vi "Main.vi"(7 "error in (no error)":errorcluster, 10 "ModuleAdmin":refnum<class "ModuleAdmin.lvclass">) -> ()   [LabVIEW 2018, in "AcPwrPlugins.lvlib"]
doc: "This VI is the critical engine of the AcPwr Plugin. It makes all the initialize, configure, and etc calls to the instrument drivers using their specifica API functions based upon the loaded configuration file."
uses:
  AcPwrPlugins/AcPwrPlugins.lvlib
  <userlib>/NIST/ModuleAdminLib/ModuleAdmin/ModuleAdmin.lvclass
  C:/Program Files (x86)/National Instruments/LabVIEW 2018/user.lib/NIST/ModuleAdminLib/ModuleAdminBase/ModuleAdminBase.lvclass
  AcPwrPlugins/AcPwrBaseClass/AcPwrBase.lvclass
  C:/Program Files (x86)/National Instruments/LabVIEW 2018/user.lib/NIST/BaseClasses/BasePlugin_class/BasePlugin.lvclass
  PublicAPI/Arguments/Requests/clStopArgument.ctl
  <userlib>/NIST/ModuleAdminLib/ModuleAdmin/ModuleAdmin.lvclass/ModuleAdmin.ctl
  <userlib>/NIST/BaseClasses/BasePlugin_class/BasePlugin.lvclass/BasePlugin.ctl
  <vilib>/Utility/error.llb/DialogType.ctl
  <userlib>/NIST/ModuleAdminLib/ModuleAdmin/Accessors/Read ShowPanel_.vi
  <userlib>/NIST/ModuleAdminLib/ModuleAdmin/Accessors/Write ShowPanel_.vi
  <userlib>/NIST/BaseClasses/BasePlugin_class/Accessors/Write PluginIniFilePath.vi
  <userlib>/NIST/BaseClasses/BasePlugin_class/Accessors/Read PluginIniFilePath.vi
  <userlib>/NIST/ModuleAdminLib/ModuleAdmin/Accessors/Read CloneRegRef.vi
  <extravilib>/ChannelInstances/Tag-bool/Read With Abort.vi
  <extravilib>/ChannelInstances/Tag-bool/Write With Abort.vi
  <extravilib>/ChannelInstances/Tag-bool/Instantiate.vi
  <extravilib>/ChannelInstances/Tag-bool/EndpointRead.vi
  <vilib>/Utility/error.llb/Error Cluster From Error Code.vi
  <extravilib>/ChannelInstances/Tag-bool/Endpoint.vi
  <vilib>/ErrorRing/Error Ring.xnode
  <userlib>/NIST/ModuleAdminLib/CloneRegistration/CloneRegistration.lvclass
  AcPwrModule.lvlib
  <userlib>/NIST/BaseClasses/Object_class/BaseObject.lvclass
  <userlib>/NIST/ModuleAdminLib/ModuleAdmin.lvlib
  <extravilib>/ChannelInstances/Tag-bool.lvlib
panel:
  out "RunTime(ms)":u32
  out "error out":errorcluster
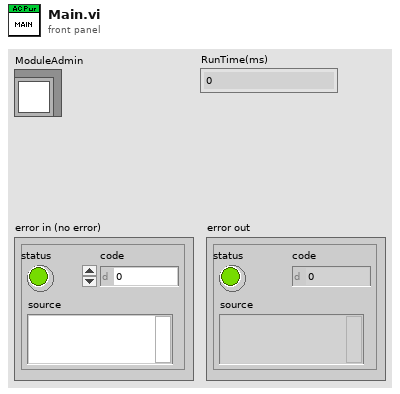
[diagram p1: front panel]
types:
  T1 = typedef "clRequestEvents.ctl" = cluster{"StopRequest":refnum<user-event>, "PathToINI":refnum<user-event>, " LoadPlugin":refnum<user-event>, "ShowPanel":refnum<user-event>, "PrefDlg":refnum<user-event>, "InitAcPwr":refnum<user-event>, "Reset":refnum<user-event>, "Close":refnum<user-event>, "StopMeas":refnum<user-event>, "StartMeas":refnum<user-event>, "ConfigDevice":refnum<user-event>, "DeviceOn":refnum<user-event>, "DeviceOff":refnum<user-event>, "GetSettings":refnum<user-event>, "SetSettings":refnum<user-event>}
  T2 = typedef "clBroadcastEvents.ctl" = cluster{"DidInit":refnum<user-event>, "StatusUpdate":refnum<user-event>, "ErrorReport":refnum<user-event>, "DidStop":refnum<user-event>, "PathToINI":refnum<user-event>, "Measurements":refnum<user-event>, "LoadConfigFile":refnum<user-event>, "GetSettings":refnum<user-event>, "SetSettings":refnum<user-event>, "GetType&ID":refnum<user-event>, "GotSettings":refnum<user-event>}
  T3 = typedef "clStopArgument.ctl" = cluster{"Exit via Stop Module Req?":bool, "Wait for Module to stop?":bool, "ModuleAdmin":refnum<class "ModuleAdmin.lvclass">}
  T4 = enum32{"Invalid", "Standard", "Closed", "Hidden", "Minimized", "Maximized"}
  T5 = typedef "Tag-bool.lvlib/))Channel.ctl" = refnum<queue>
  T6 = typedef "DialogType.ctl" = u16
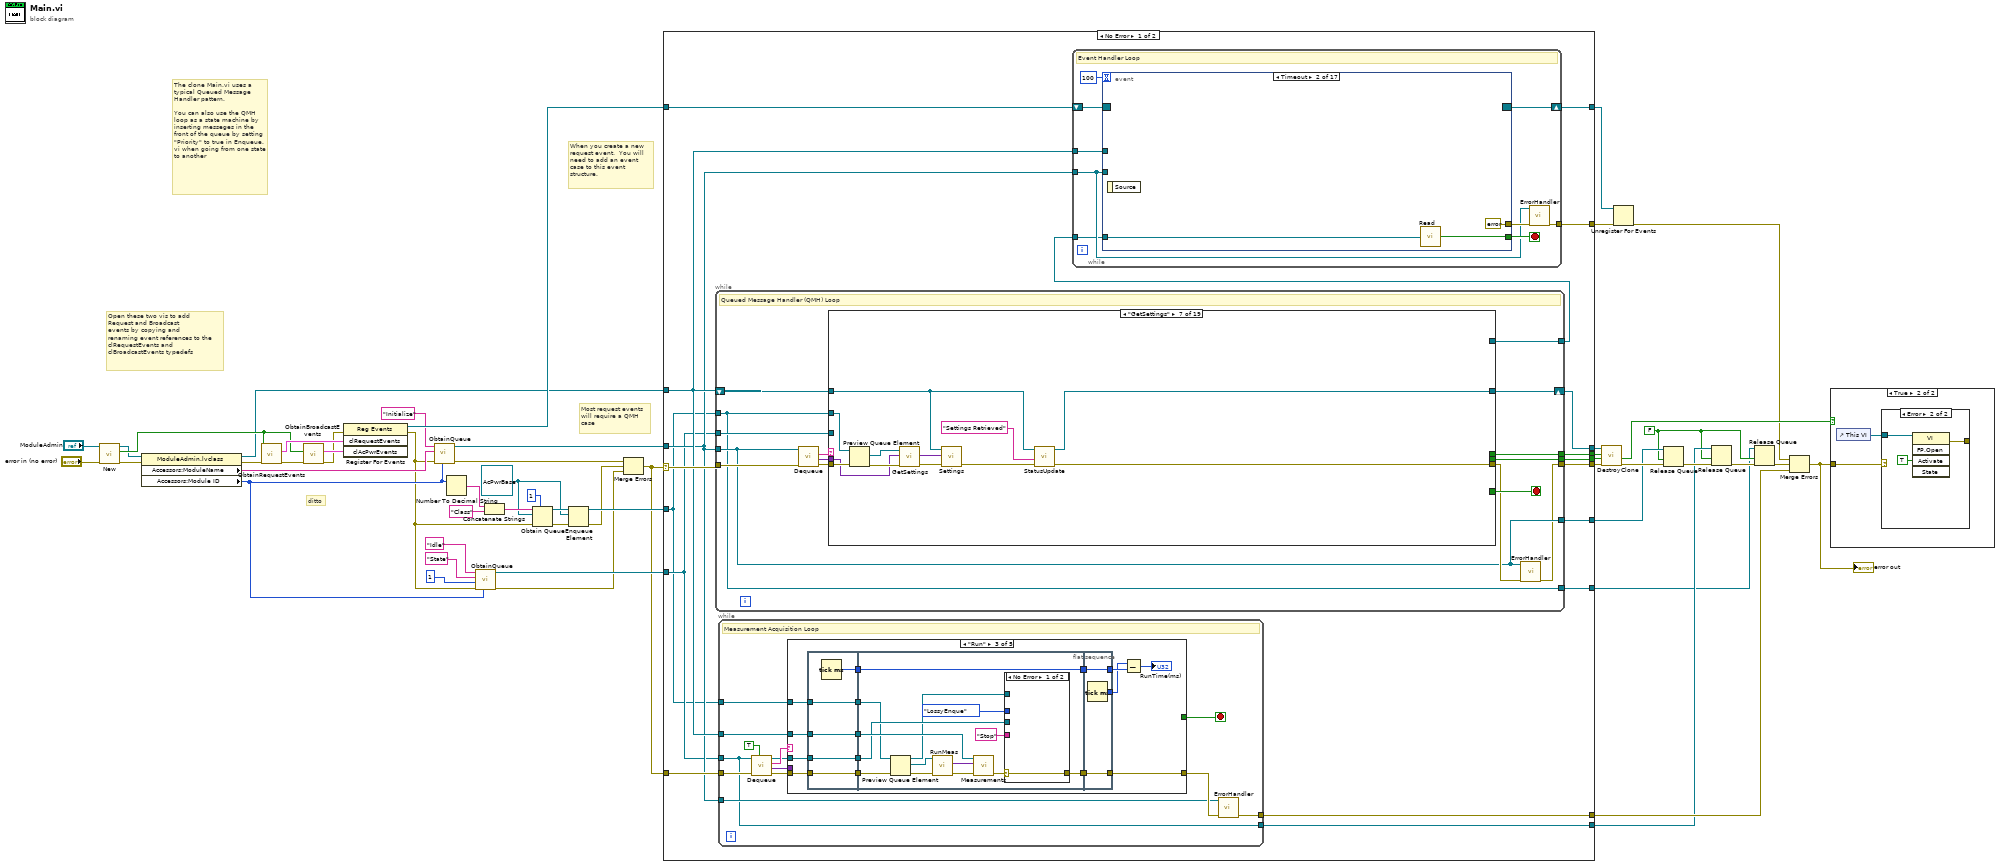
[diagram p0: block diagram]
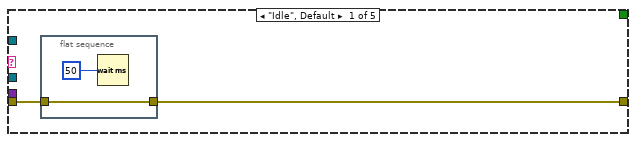
[diagram p2: hidden frame]
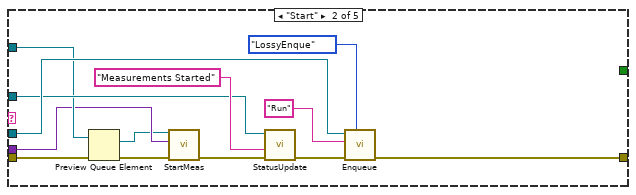
[diagram p3: hidden frame]
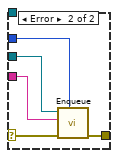
[diagram p4: hidden frame]
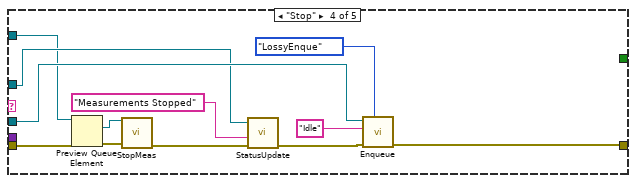
[diagram p5: hidden frame]
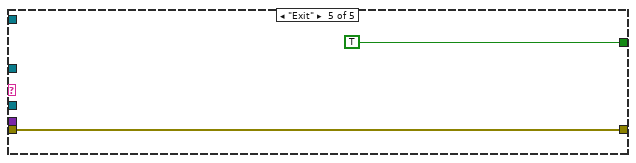
[diagram p6: hidden frame]
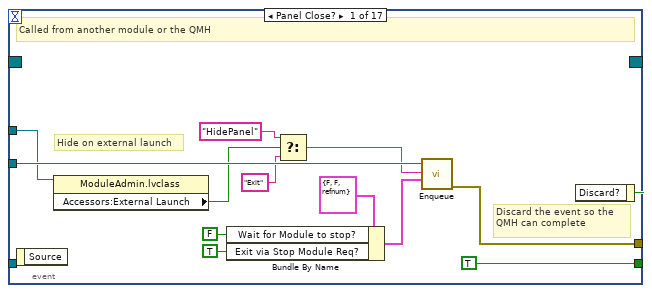
[diagram p7: hidden frame]
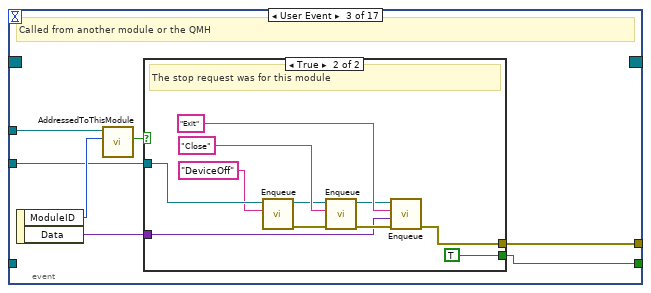
[diagram p8: hidden frame]
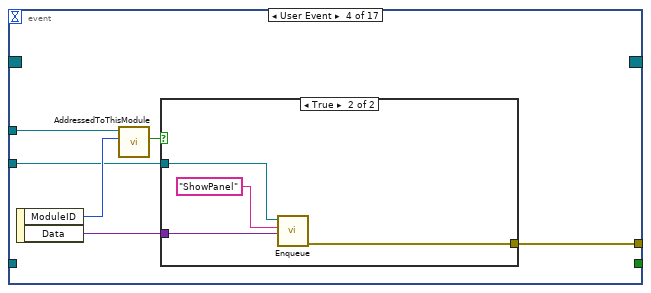
[diagram p10: hidden frame]
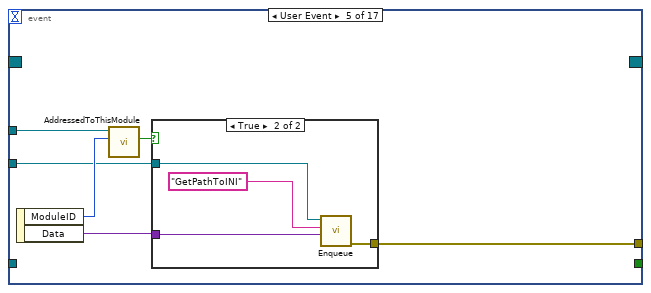
[diagram p12: hidden frame]
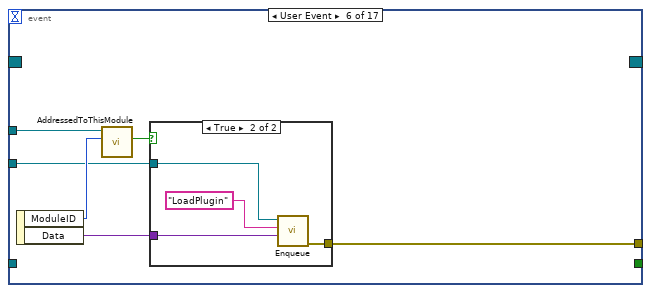
[diagram p14: hidden frame]
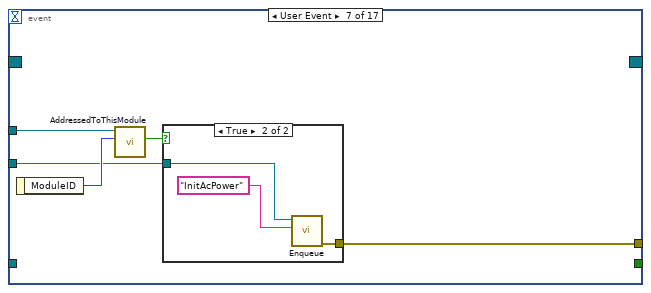
[diagram p16: hidden frame]
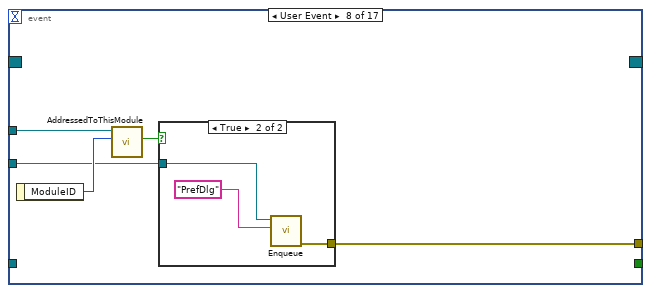
[diagram p18: hidden frame]
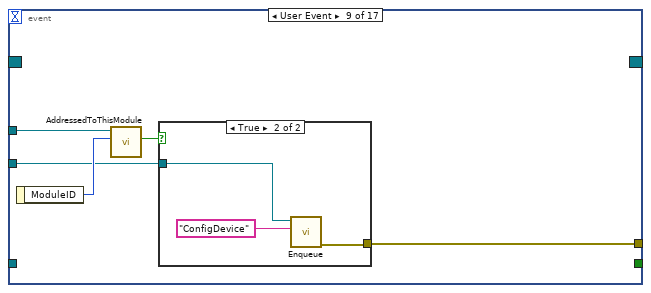
[diagram p20: hidden frame]
diagram:
  w13 = refnum<class "AcPwrBase.lvclass"> refnum ("MyPlugins.lvlib:MyPluginsBase.lvclass")
  w19 = FALSE ("force destroy? (F)")
  # "The clone Main.vi uses a typical Queued Message Handler pattern.  \n\nYou can also use the QMH loop as a state machine by inserting messeges in the front of the queue by setting \"Priority\" to true in Enqueue.vi when going from one state to another"
  # "Open these two vis to add\nRequest and Broadcast \nevents by copying and \nrenaming event references to the \nclRequestEvents and \nclBroadcastEvents typedefs"
  # "ditto"
  # "Most request events\nwill require a QMH\ncase"
  # "When you create a new request event.  You will need to add an event case to this event structure."
  n1 = call <userlib>:"New.vi"("error in (no error)"="error in (no error)", "ModuleAdmin"="ModuleAdmin") -> ("error out"=w33:errorcluster, "First?"=w47:bool, "ModuleAdmin"=w34:refnum<class "ModuleAdmin.lvclass">)  [unwired: 6 in, 1 out]
  n2 = property class="ModuleAdmin.lvclass"(reference=w34, error in=w33) -> (reference out=w30:refnum<class "ModuleAdmin.lvclass">, error out=w32:errorcluster, "Accessors:ModuleName"=w31:string, "Accessors:Module ID"=w23:i32)
  n3 = call "ObtainRequestEvents.vi"("error in (no error)"=w32, "CreateNew (F)"=w47) -> ("error out"=w46:errorcluster, "clRequestEvents"=w49:T1)  [unwired: 8 in]
  n4 = call "ObtainBroadcastEvents.vi"("error in (no error)"=w46, "CreateNew? (F)"=w47) -> ("error out"=w12:errorcluster, "clAcPwrEvents"=w45:T2)  [unwired: 8 in]
  n5 = register-events(error in=w12, w49, w45) -> (reference out=w44:refnum<event-registration>, error out=w11:errorcluster)  [unwired: 1 in]
  n6 = call "ObtainQueue.vi"("ModuleID"=w23, "error in (no error)"=w11, "ModuleName"=w31, "Initial Message"="Initialize" ("ModuleName")) -> ("error out"=w7:errorcluster, "MessageQueue"=w48:refnum<queue>)  [unwired: 6 in]
  n7 = Number To Decimal String(number=w23) -> (decimal integer string=w24:string)  [unwired: 1 in]
  n8 = call "ObtainQueue.vi"("ModuleID"=w23, "error in (no error)"=w11, "max queue size (-1, unlimited)"=1, "ModuleName"="State", "Initial Message"="Idle") -> ("error out"=w5:errorcluster, "MessageQueue"=w28:refnum<queue>)  [unwired: 5 in]
  n9 = Concatenate Strings(w24, "Class" ("ModuleName")) -> (w21:string)
  n10 = Obtain Queue(max queue size (-1, unlimited)=1, name (unnamed)=w21, element data type=w13, error in (no error)=w11) -> (queue out=w15:refnum<queue>, error out=w20:errorcluster)  [unwired: 1 in, 1 out]
  n11 = Enqueue Element(queue=w15, element=w13, error in (no error)=w20) -> (queue out=w14:refnum<queue>, error out=w6:errorcluster)  [unwired: 1 in, 1 out]
  n12 = Merge Errors(w7, w6, w5) -> (w4:errorcluster)
  n13 = case shown="No Error" w4 {
    selector: w4 -> [w69 w920]
    tunnel: w48 -> [w57 w913]
    tunnel: w30 -> [w58 w918]
    tunnel: [w68 w909] -> w1
    tunnel: w44 -> [w67 w914]
    tunnel: [w66 w917] -> w2
    tunnel: [w65 _] -> w42
    tunnel: [w64 _] -> w41
    tunnel: [w63 w909] -> w39
    tunnel: [w62 w914] -> w38
    tunnel: [w61 w913] -> w35
    tunnel: w4 -> [w60 w912]
    tunnel: [w59 w912] -> w29
    tunnel: w28 -> [w55 w911]
    tunnel: [w56 w911] -> w26
    tunnel: w14 -> [w54 w910]
    tunnel: [w53 w910] -> w16
    frame No Error {
      n14 = while {
        tunnel: w57 -> [w339]
        tunnel: w69 -> [w348]
        tunnel: [w338] -> w68
        tunnel: [w343] -> w65
        tunnel: [w342] -> w64
        shift-right: [w340] -> w66
        shift-left: w58 -> [w344]
        tunnel: [w339] -> w61
        tunnel: w55 -> [w337]
        tunnel: w54 -> [w336]
        tunnel: [w336] -> w53
        tunnel: [w335] -> w52
        stop <- w349 stop-if-true
        # "Queued Message Handler (QMH) Loop"
        n15 = call "Dequeue.vi"("error in (no error)"=w348, "MessageQueue"=w339) -> ("error out"=w347:errorcluster, "Message Data"=w345:variant, "Message"=w346:string)  [unwired: 5 in, 2 out]
        n16 = case shown="\"GetSettings\"" w346 {
          selector: w346 -> [_ _ _ _ _ _ _ _ _ _ _ _ _ _ _ _ _ _ w897]
          tunnel: [_ _ _ _ _ _ _ _ _ _ _ _ _ _ _ _ w857 _ _] -> w349
          tunnel: w344 -> [w371 w388 w395 w447 w460 w491 w533 w556 w611 w620 w668 w715 w721 w731 w826 w849 w860 w874 w900]
          tunnel: [w360 w382 w396 w448 w459 w490 w539 w555 w601 w622 w671 w716 w722 w732 w828 w850 w868 w875 w892] -> w341
          tunnel: w347 -> [w353 w391 w405 w442 w456 w489 w543 w554 w607 w618 w667 w717 w723 w727 w815 w837 w864 w872 _]
          tunnel: w345 -> [_ w390 w407 _ _ _ w532 w544 _ _ _ w711 _ _ _ _ w861 w882 _]
          tunnel: [_ _ _ _ _ _ _ _ _ _ _ _ _ _ _ _ w866 _ _] -> w343
          tunnel: [_ _ _ _ _ _ _ _ _ _ _ _ _ _ _ _ w865 _ _] -> w342
          tunnel: [w354 w387 w393 w446 w458 w486 w537 w551 w600 w619 w669 w715 w721 w730 w825 w848 w860 w873 w895] -> w340
          tunnel: w337 -> [_ _ _ _ w454 w485 _ w550 w599 w621 w670 w714 w720 w728 w813 w840 w862 _ _]
          tunnel: w336 -> [_ _ w392 w440 w453 w488 w542 w553 _ w617 w666 _ _ w724 w816 w835 _ _ _]
          tunnel: [_ _ _ _ _ _ _ _ _ _ _ _ _ _ _ _ w856 w871 _] -> w335
          frame "Initialize" {
            # "After the QMH, Class, and State Queue have been created this loop enters the intialize phase."
            n17 = property class="ModuleAdmin.lvclass"(reference=w371, error in=w353) -> (reference out=w358:refnum<class "ModuleAdmin.lvclass">, error out=w368:errorcluster, "Accessors:ShowPanel_"=w357:bool, "Accessors:External Launch"=w356:bool, "Accessors:Module ID"=w351:i32, "Accessors:ModuleName"=w352:string)
            n18 = Compound Arithmetic op=OR(w357, invert w356) -> (w355:bool)
            n19 = Select(t=T4."Standard" ("Front Panel Window:State"), s=w355, f=T4."Hidden" ("Front Panel Window:State")) -> (s? t:f=w364:T4)
            n20 = invoke class="VI" method="FP.Open"(error in=w368, "State"=w364) -> (reference out=w350:refnum<vi>, error out=w367:errorcluster)  [unwired: 3 in, 3 out]
            n21 = call <userlib>:"ModuleName.vi"("Name"=w352, "ModuleID"=w351) -> ("ModuleName"=w363:string)  [unwired: 9 in]
            n22 = property class="VI"(reference=w350, error in=w367, "Front Panel.Title"=w363) -> (reference out=w370:refnum<vi>, error out=w369:errorcluster)
            n23 = invoke class="VI" method="FP.Center"(reference=w370, error in=w369) -> (error out=w359:errorcluster)  [unwired: 1 in, 2 out]
            n24 = case shown="True" w356 {
              tunnel: [w372 w378] -> w361
              tunnel: [w373 w375] -> w354
              tunnel: w359 -> [w372 w377]
              tunnel: w358 -> [w373 w374]
              frame False {
              }
              frame True {
                n25 = call <userlib>:"WaitOnModuleSync.vi"("error in (no error)"=w377, "ModuleAdmin"=w374) -> ("error out"=w379:errorcluster, "ModuleAdmin"=w376:refnum<class "ModuleAdmin.lvclass">)  [unwired: 8 in]
                n26 = call <userlib>:"WaitOnEventSync.vi"("error in (no error)"=w379, "ModuleAdmin"=w376) -> ("error out"=w378:errorcluster, "ModuleAdmin"=w375:refnum<class "ModuleAdmin.lvclass">)  [unwired: 8 in]
              }
            }
            n27 = call "DidInit.vi"("Init?"=TRUE, "error in (no error)"=w361, "ModuleAdmin"=w354) -> ("error out"=w360:errorcluster)  [unwired: 8 in]
          }
          frame "ShowPanel" {
            # "The front panel can be shown or hidden"
            n28 = Variant To Data(error in=w391, type=TRUE, Variant=w390) -> (data=w384:bool, error out=w381:errorcluster)
            n29 = property class="ModuleAdmin.lvclass"(reference=w388, error in=w381, "Accessors:ShowPanel_"=w384) -> (reference out=w387:refnum<class "ModuleAdmin.lvclass">, error out=w380:errorcluster)
            n30 = Select(t=T4."Standard" ("Front Panel Window:State"), s=w384, f=T4."Hidden" ("Front Panel Window:State")) -> (s? t:f=w383:T4)
            n31 = property class="VI"(error in=w380, "FP.State"=w383) -> (error out=w382:errorcluster)  [unwired: 1 in, 1 out]
          }
          frame "LoadPlugin" {
            # "Dynamically oads and initializes a plugin from the .ini file"
            n32 = Variant To Data(error in=w405, type=path "", Variant=w407) -> (data=w394:path, error out=w404:errorcluster)
            n33 = Current VI's Path() -> (path=w402:path)
            n34 = call <userlib>:"GetPathToClass.vi"("error in (no error)"=w404, "configuration file path"=w394) -> ("error IO"=w400:errorcluster, "PathToClass"=w403:path)  [unwired: 8 in]
            n35 = Build Path(base path=w402, name or relative path=w403) -> (appended path=w401:path)
            n36 = call <vilib>:"Check if File or Folder Exists.vi"("error in (no error)"=w400, "path"=w401) -> ("error out"=w397:errorcluster, "file or folder exists?"=w399:bool, "dup path"=w398:path)  [unwired: 7 in]
            n37 = case shown="False" w399 {
              tunnel: w398 -> [w410 w419]
              tunnel: w397 -> [_ w426]
              tunnel: [w409 w436] -> w396
              tunnel: w395 -> [w408 w432]
              tunnel: w394 -> [_ w433]
              tunnel: [w408 w431] -> w393
              tunnel: w392 -> [_ w424]
              frame False {
                n38 = Path To String(path=w410) -> (string=w411:string)
                n39 = xnode "Error Ring"("parameter 0"=w411) -> ("error out"=w409:errorcluster)
              }
              frame True {
                (unwired) refnum<class "AcPwrBase.lvclass"> refnum ("MyPlugins.lvlib:MyPluginsBase.lvclass")
                n40 = Strip Path(path=w419) -> (name=w422:string)  [unwired: 1 out]
                n41 = Preview Queue Element(queue=w424, error in (no error)=w426) -> (element=w423:refnum<class "AcPwrBase.lvclass">, error out=w425:errorcluster)  [unwired: 1 in, 2 out]
                n42 = call-dynamic "LoadClassFromFile.vi"("error in (no error)"=w425, "class path"=w419, "reference in"=w423) -> ("error out"=w434:errorcluster, "reference out"=w435:refnum<class "AcPwrBase.lvclass">)  [unwired: 7 in]
                n43 = property class="AcPwrBase.lvclass"(reference=w435, error in=w434, "Accessors:PluginIniFilePath"=w433) -> (reference out=w430:refnum<class "AcPwrBase.lvclass">, error out=w429:errorcluster)
                n44 = call-dynamic "DefaultFromIni.vi"("error in (no error)"=w429, "AcPwrBase"=w430) -> ("error out"=w427:errorcluster, "AcPwrBase"=w428:refnum<class "AcPwrBase.lvclass">)  [unwired: 8 in]
                n45 = Lossy Enqueue Element(queue=w424, element=w428, error in (no error)=w427) -> (error out=w420:errorcluster)  [unwired: 3 out]
                n46 = Format Into String(format string="Plugin %s loaded ", error in=w420, w422) -> (resulting string=w437:string, error out=w421:errorcluster)  [unwired: 1 in]
                n47 = call "StatusUpdate.vi"("error in (no error)"=w421, "Status"=w437, "Module"=w432) -> ("error out"=w436:errorcluster, "Module"=w431:refnum<class "ModuleAdmin.lvclass">)  [unwired: 7 in]
              }
            }
          }
          frame "GetPathToINI" {
            # "Broadcast the path to the .ini file"
            n48 = Preview Queue Element(queue=w440, error in (no error)=w442) -> (element=w445:refnum<class "AcPwrBase.lvclass">, error out=w441:errorcluster)  [unwired: 1 in, 2 out]
            n49 = property class="AcPwrBase.lvclass"(reference=w445, error in=w441) -> (error out=w444:errorcluster, "Accessors:PluginIniFilePath"=w439:path)  [unwired: 1 out]
            n50 = property class="ModuleAdmin.lvclass"(reference=w447, error in=w444) -> (reference out=w446:refnum<class "ModuleAdmin.lvclass">, error out=w443:errorcluster, "Accessors:Module ID"=w449:i32)
            n51 = call "PathToINIBroadcast.vi"("error in (no error)"=w443, "PathToINI"=w439, "ModuleID"=w449) -> ("error out"=w448:errorcluster)  [unwired: 8 in]
          }
          frame "InitAcPower" {
            n52 = call "Dequeue.vi"("PreviewQueue(F)"=TRUE, "error in (no error)"=w456, "MessageQueue"=w454) -> ("error out"=w455:errorcluster, "Message"=w451:string)  [unwired: 4 in, 3 out]
            n53 = Equal?(x="Run" ("y"), y=w451) -> (x = y?=w457:bool)
            n54 = case shown="False" w457 {
              tunnel: w460 -> [w472 w474]
              tunnel: [w471 w473] -> w459
              tunnel: [w469 w474] -> w458
              tunnel: w455 -> [w466 _]
              tunnel: w453 -> [w464 _]
              frame False {
                n55 = Preview Queue Element(queue=w464, error in (no error)=w466) -> (queue out=w462:refnum<queue>, element=w468:refnum<class "AcPwrBase.lvclass">, error out=w465:errorcluster)  [unwired: 1 in, 1 out]
                n56 = call-dynamic "Initialize.vi"("error in (no error)"=w465, "AcPwrBase in"=w468) -> ("error out"=w463:errorcluster, "AcPwrBase out"=w467:refnum<class "AcPwrBase.lvclass">)  [unwired: 8 in]
                n57 = Lossy Enqueue Element(queue=w462, element=w467, error in (no error)=w463) -> (error out=w461:errorcluster)  [unwired: 3 out]
                n58 = call "StatusUpdate.vi"("error in (no error)"=w461, "Status"="Device Initialized", "Module"=w472) -> ("error out"=w471:errorcluster, "Module"=w469:refnum<class "ModuleAdmin.lvclass">)  [unwired: 7 in]
              }
              frame True {
                n59 = xnode "Error Ring"() -> ("error out"=w473:errorcluster)
              }
            }
          }
          frame "ConfigDevice" {
            n60 = Preview Queue Element(queue=w488, error in (no error)=w489) -> (queue out=w487:refnum<queue>, element=w483:refnum<class "AcPwrBase.lvclass">, error out=w484:errorcluster)  [unwired: 1 in, 1 out]
            n61 = call-dynamic "ChangeWhileMeasuring.vi"("error in (no error)"=w484, "AcPwrBase in"=w483) -> ("error out"=w482:errorcluster, "OutputOrLoadValue"=w480:bool, "AcPwrBase out"=w481:refnum<class "AcPwrBase.lvclass">)  [unwired: 6 in, 1 out]
            n62 = case shown="True" w480 {
              tunnel: w491 -> [w501 w526]
              tunnel: w481 -> [w499 w508]
              tunnel: [w498 w518] -> w490
              tunnel: w482 -> [w497 w511]
              tunnel: w487 -> [w493 w515]
              tunnel: [w496 w514] -> w486
              tunnel: w485 -> [_ w510]
              frame True {
                n63 = call-dynamic "ConfigDevice.vi"("error in (no error)"=w497, "AcPwrBase in"=w499) -> ("error out"=w495:errorcluster, "AcPwrBase out"=w492:refnum<class "AcPwrBase.lvclass">)  [unwired: 8 in]
                n64 = Lossy Enqueue Element(queue=w493, element=w492, error in (no error)=w495) -> (error out=w494:errorcluster)  [unwired: 3 out]
                n65 = call "StatusUpdate.vi"("error in (no error)"=w494, "Status"="Device Configured", "Module"=w501) -> ("error out"=w498:errorcluster, "Module"=w496:refnum<class "ModuleAdmin.lvclass">)  [unwired: 7 in]
              }
              frame False {
                w523 = TRUE ("OverwriteClass? (F)")
                n66 = call "Dequeue.vi"("PreviewQueue(F)"=TRUE, "error in (no error)"=w511, "MessageQueue"=w510) -> ("error out"=w509:errorcluster, "Message"=w503:string, "MessageQueue"=w502:refnum<queue>)  [unwired: 4 in, 2 out]
                n67 = Equal?(x="Run" ("y"), y=w503) -> (x = y?=w506:bool)
                n68 = call "CheckonIdle.vi"("MessageQueue"=w502, "OverwriteClass? (F)"=w523, "error in (no error)"=w509, "ChangeOccured? (F)"=w523, "AcPwrBase in"=w508) -> ("Error Out"=w524:errorcluster, "Write?"=w520:bool, "AcPwrBase out"=w522:refnum<class "AcPwrBase.lvclass">)  [unwired: 4 in]
                n69 = call-dynamic "ConfigDevice.vi"("error in (no error)"=w524, "AcPwrBase in"=w522) -> ("error out"=w517:errorcluster, "AcPwrBase out"=w521:refnum<class "AcPwrBase.lvclass">)  [unwired: 8 in]
                n70 = case shown="True" w520 {
                  tunnel: [w527 w531] -> w516
                  tunnel: w517 -> [w527 w530]
                  tunnel: w515 -> [_ w529]
                  tunnel: w521 -> [_ w528]
                  frame False {
                  }
                  frame True {
                    n71 = Lossy Enqueue Element(queue=w529, element=w528, error in (no error)=w530) -> (error out=w531:errorcluster)  [unwired: 3 out]
                  }
                }
                n72 = call "StatusUpdate.vi"("error in (no error)"=w516, "Status"="Device Configured", "Module"=w526) -> ("error out"=w519:errorcluster, "Module"=w514:refnum<class "ModuleAdmin.lvclass">)  [unwired: 7 in]
                n73 = Select(t="Start" ("strngStateIn"), s=w506, f=w503) -> (s? t:f=w504:string)
                n74 = call "Enqueue.vi"("EnqueType (Enque)"=enum16{"LossyEnque", "EnqueAtFront", "Enque"}."LossyEnque" ("Enum"), "error in (no error)"=w519, "Message"=w504, "MessageQueue"=w502) -> ("error out"=w518:errorcluster)  [unwired: 6 in, 1 out]
              }
            }
          }
          frame "GetSettings" {
            n75 = Preview Queue Element(queue=w542, error in (no error)=w543) -> (element=w540:refnum<class "AcPwrBase.lvclass">, error out=w541:errorcluster)  [unwired: 1 in, 2 out]
            n76 = call-dynamic "GetSettings.vi"("error in (no error)"=w541, "SettingsToRetrieve"=w532, "AcPwrBase in"=w540) -> ("error out"=w536:errorcluster, "RetrievedSettings"=w534:variant)  [unwired: 6 in, 1 out]
            n77 = call "Settings.vi"("error in (no error)"=w536, "variant"=w534, "Module"=w533) -> ("error out"=w535:errorcluster)  [unwired: 8 in]
            n78 = call "StatusUpdate.vi"("error in (no error)"=w535, "Status"="Settings Retrieved", "Module"=w533) -> ("error out"=w539:errorcluster, "Module"=w537:refnum<class "ModuleAdmin.lvclass">)  [unwired: 7 in]
          }
          frame "SetSettings" {
            n79 = Preview Queue Element(queue=w553, error in (no error)=w554) -> (queue out=w552:refnum<queue>, element=w548:refnum<class "AcPwrBase.lvclass">, error out=w549:errorcluster)  [unwired: 1 in, 1 out]
            n80 = call-dynamic "ChangeWhileMeasuring.vi"("error in (no error)"=w549, "AcPwrBase in"=w548) -> ("error out"=w547:errorcluster, "OutputOrLoadValue"=w545:bool, "AcPwrBase out"=w546:refnum<class "AcPwrBase.lvclass">)  [unwired: 6 in, 1 out]
            n81 = case shown="True" w545 {
              tunnel: w556 -> [w567 w593]
              tunnel: w546 -> [w560 w570]
              tunnel: [w565 w588] -> w555
              tunnel: w547 -> [w561 w582]
              tunnel: w552 -> [w562 w586]
              tunnel: [w564 w585] -> w551
              tunnel: w550 -> [_ w581]
              tunnel: w544 -> [w559 w571]
              frame True {
                n82 = call-dynamic "SetSettings.vi"("error in (no error)"=w561, "Variant"=w559, "AcPwrBase in"=w560) -> ("error out"=w557:errorcluster, "AcPwrBase Out"=w558:refnum<class "AcPwrBase.lvclass">)  [unwired: 7 in]
                n83 = Lossy Enqueue Element(queue=w562, element=w558, error in (no error)=w557) -> (error out=w563:errorcluster)  [unwired: 3 out]
                n84 = call "StatusUpdate.vi"("error in (no error)"=w563, "Status"="Settings Set", "Module"=w567) -> ("error out"=w565:errorcluster, "Module"=w564:refnum<class "ModuleAdmin.lvclass">)  [unwired: 7 in]
              }
              frame False {
                w591 = TRUE ("OverwriteClass? (F)")
                n85 = call "Dequeue.vi"("PreviewQueue(F)"=TRUE, "error in (no error)"=w582, "MessageQueue"=w581) -> ("error out"=w580:errorcluster, "Message"=w575:string, "MessageQueue"=w574:refnum<queue>)  [unwired: 4 in, 2 out]
                n86 = Equal?(x="Run" ("y"), y=w575) -> (x = y?=w578:bool)
                n87 = call "CheckonIdle.vi"("MessageQueue"=w574, "OverwriteClass? (F)"=w591, "error in (no error)"=w580, "ChangeOccured? (F)"=w591, "AcPwrBase in"=w570) -> ("Error Out"=w572:errorcluster, "Write?"=w590:bool, "AcPwrBase out"=w573:refnum<class "AcPwrBase.lvclass">)  [unwired: 4 in]
                n88 = call-dynamic "SetSettings.vi"("error in (no error)"=w572, "Variant"=w571, "AcPwrBase in"=w573) -> ("error out"=w568:errorcluster, "AcPwrBase Out"=w569:refnum<class "AcPwrBase.lvclass">)  [unwired: 7 in]
                n89 = Select(t="Start" ("strngStateIn"), s=w578, f=w575) -> (s? t:f=w576:string)
                n90 = case shown="True" w590 {
                  tunnel: [w594 w598] -> w587
                  tunnel: w568 -> [w594 w597]
                  tunnel: w586 -> [_ w596]
                  tunnel: w569 -> [_ w595]
                  frame False {
                  }
                  frame True {
                    n91 = Lossy Enqueue Element(queue=w596, element=w595, error in (no error)=w597) -> (error out=w598:errorcluster)  [unwired: 3 out]
                  }
                }
                n92 = call "StatusUpdate.vi"("error in (no error)"=w587, "Status"="Settings Set", "Module"=w593) -> ("error out"=w589:errorcluster, "Module"=w585:refnum<class "ModuleAdmin.lvclass">)  [unwired: 7 in]
                n93 = call "Enqueue.vi"("EnqueType (Enque)"=enum16{"LossyEnque", "EnqueAtFront", "Enque"}."LossyEnque" ("Enum"), "error in (no error)"=w589, "Message"=w576, "MessageQueue"=w574) -> ("error out"=w588:errorcluster)  [unwired: 6 in, 1 out]
              }
            }
          }
          frame "ConfigPhase" {
            w605 = TRUE ("btnSet")
            # "Need to figure out if this case is really needed or can be put into config device."
            n94 = call "AcPwrClass.vi"() -> ("Class Out"=w606:refnum<class "AcPwrBase.lvclass">)  [unwired: 11 in]
            n95 = call "CheckonIdle.vi"("MessageQueue"=w599, "OverwriteClass? (F)"=w605, "error in (no error)"=w607, "ChangeOccured? (F)"=w605, "AcPwrBase in"=w606) -> ("Error Out"=w604:errorcluster, "Write?"=w602:bool, "AcPwrBase out"=w603:refnum<class "AcPwrBase.lvclass">)  [unwired: 4 in]
            n96 = call-dynamic "ConfigPhases.vi"("error in (no error)"=w604, "AcPwrBase in"=w603) -> ("error out"=w608:errorcluster, "AcPwrBase out"=w609:refnum<class "AcPwrBase.lvclass">)  [unwired: 8 in]
            n97 = call "AcPwrClass.vi"("btnSet"=w602, "Class In"=w609) -> ()  [unwired: 9 in, 1 out]
            n98 = call "StatusUpdate.vi"("error in (no error)"=w608, "Status"="PhaseAngle Configured", "Module"=w611) -> ("error out"=w601:errorcluster, "Module"=w600:refnum<class "ModuleAdmin.lvclass">)  [unwired: 7 in]
          }
          frame "DeviceOn" {
            # "Turns the device on."
            n99 = Preview Queue Element(queue=w617, error in (no error)=w618) -> (element=w615:refnum<class "AcPwrBase.lvclass">, error out=w616:errorcluster)  [unwired: 1 in, 2 out]
            n100 = call-dynamic "ChangeWhileMeasuring.vi"("error in (no error)"=w616, "AcPwrBase in"=w615) -> ("error out"=w614:errorcluster, "OutputOrLoadValue"=w613:bool, "AcPwrBase out"=w612:refnum<class "AcPwrBase.lvclass">)  [unwired: 6 in, 1 out]
            n101 = case shown="False" w613 {
              tunnel: [w640 w656] -> w622
              tunnel: w621 -> [w639 _]
              tunnel: w620 -> [w623 w659]
              tunnel: w617 -> [w634 _]
              tunnel: [w629 w658] -> w619
              tunnel: w614 -> [w628 w655]
              tunnel: w612 -> [_ w654]
              frame False {
                w643 = TRUE ("OverwriteClass? (F)")
                n102 = call "Dequeue.vi"("PreviewQueue(F)"=TRUE, "error in (no error)"=w628, "MessageQueue"=w639) -> ("error out"=w638:errorcluster, "Message"=w625:string, "MessageQueue"=w626:refnum<queue>)  [unwired: 4 in, 2 out]
                n103 = Preview Queue Element(queue=w634, error in (no error)=w638) -> (element=w645:refnum<class "AcPwrBase.lvclass">, error out=w637:errorcluster)  [unwired: 1 in, 2 out]
                n104 = Equal?(x="Run" ("y"), y=w625) -> (x = y?=w627:bool)
                n105 = call "CheckonIdle.vi"("MessageQueue"=w626, "OverwriteClass? (F)"=w643, "error in (no error)"=w637, "ChangeOccured? (F)"=w643, "AcPwrBase in"=w645) -> ("Error Out"=w646:errorcluster, "Write?"=w642:bool, "AcPwrBase out"=w644:refnum<class "AcPwrBase.lvclass">)  [unwired: 4 in]
                n106 = call-dynamic "DeviceOn.vi"("error in (no error)"=w646, "AcPwrBase in"=w644) -> ("error out"=w636:errorcluster, "AcPwrBase out"=w648:refnum<class "AcPwrBase.lvclass">)  [unwired: 8 in]
                n107 = case shown="True" w642 {
                  tunnel: w636 -> [w649 w653]
                  tunnel: [w649 w652] -> w635
                  tunnel: w634 -> [_ w651]
                  tunnel: w648 -> [_ w650]
                  frame False {
                  }
                  frame True {
                    n108 = Lossy Enqueue Element(queue=w651, element=w650, error in (no error)=w653) -> (error out=w652:errorcluster)  [unwired: 3 out]
                  }
                }
                n109 = call "StatusUpdate.vi"("error in (no error)"=w635, "Status"="Device On", "Module"=w623) -> ("error out"=w641:errorcluster, "Module"=w629:refnum<class "ModuleAdmin.lvclass">)  [unwired: 7 in]
                n110 = Select(t="Start" ("strngStateIn"), s=w627, f=w625) -> (s? t:f=w632:string)
                n111 = call "Enqueue.vi"("EnqueType (Enque)"=enum16{"LossyEnque", "EnqueAtFront", "Enque"}."LossyEnque" ("Enum"), "error in (no error)"=w641, "Message"=w632, "MessageQueue"=w626) -> ("error out"=w640:errorcluster)  [unwired: 6 in, 1 out]
              }
              frame True {
                n112 = call-dynamic "DeviceOn.vi"("error in (no error)"=w655, "AcPwrBase in"=w654) -> ("error out"=w657:errorcluster)  [unwired: 8 in, 1 out]
                n113 = call "StatusUpdate.vi"("error in (no error)"=w657, "Status"="Device On", "Module"=w659) -> ("error out"=w656:errorcluster, "Module"=w658:refnum<class "ModuleAdmin.lvclass">)  [unwired: 7 in]
              }
            }
          }
          frame "DeviceOff" {
            # "Turn the instruments channel off."
            n114 = Preview Queue Element(queue=w666, error in (no error)=w667) -> (element=w664:refnum<class "AcPwrBase.lvclass">, error out=w665:errorcluster)  [unwired: 1 in, 2 out]
            n115 = call-dynamic "ChangeWhileMeasuring.vi"("error in (no error)"=w665, "AcPwrBase in"=w664) -> ("error out"=w663:errorcluster, "OutputOrLoadValue"=w661:bool, "AcPwrBase out"=w662:refnum<class "AcPwrBase.lvclass">)  [unwired: 6 in, 1 out]
            n116 = case shown="False" w661 {
              tunnel: [w676 w697] -> w671
              tunnel: w670 -> [_ w695]
              tunnel: [w677 w693] -> w669
              tunnel: w668 -> [w673 w686]
              tunnel: w663 -> [w675 w680]
              tunnel: w666 -> [_ w679]
              tunnel: w662 -> [w674 _]
              frame True {
                n117 = call-dynamic "DeviceOff.vi"("error in (no error)"=w675, "AcPwrBase in"=w674) -> ("error out"=w672:errorcluster)  [unwired: 8 in, 1 out]
                n118 = call "StatusUpdate.vi"("error in (no error)"=w672, "Status"="Device Off", "Module"=w673) -> ("error out"=w676:errorcluster, "Module"=w677:refnum<class "ModuleAdmin.lvclass">)  [unwired: 7 in]
              }
              frame False {
                w702 = TRUE ("OverwriteClass? (F)")
                n119 = call "Dequeue.vi"("PreviewQueue(F)"=TRUE, "error in (no error)"=w680, "MessageQueue"=w695) -> ("error out"=w692:errorcluster, "Message"=w694:string, "MessageQueue"=w690:refnum<queue>)  [unwired: 4 in, 2 out]
                n120 = Preview Queue Element(queue=w679, error in (no error)=w692) -> (queue out=w687:refnum<queue>, element=w703:refnum<class "AcPwrBase.lvclass">, error out=w691:errorcluster)  [unwired: 1 in, 1 out]
                n121 = Equal?(x="Run" ("y"), y=w694) -> (x = y?=w696:bool)
                n122 = call "CheckonIdle.vi"("MessageQueue"=w690, "OverwriteClass? (F)"=w702, "error in (no error)"=w691, "ChangeOccured? (F)"=w702, "AcPwrBase in"=w703) -> ("Error Out"=w701:errorcluster, "Write?"=w699:bool, "AcPwrBase out"=w700:refnum<class "AcPwrBase.lvclass">)  [unwired: 4 in]
                n123 = call-dynamic "DeviceOff.vi"("error in (no error)"=w701, "AcPwrBase in"=w700) -> ("error out"=w689:errorcluster, "AcPwrBase out"=w704:refnum<class "AcPwrBase.lvclass">)  [unwired: 8 in]
                n124 = case shown="True" w699 {
                  tunnel: w689 -> [w706 w710]
                  tunnel: w704 -> [_ w709]
                  tunnel: [w706 w708] -> w688
                  tunnel: w687 -> [_ w707]
                  frame False {
                  }
                  frame True {
                    n125 = Lossy Enqueue Element(queue=w707, element=w709, error in (no error)=w710) -> (error out=w708:errorcluster)  [unwired: 3 out]
                  }
                }
                n126 = call "StatusUpdate.vi"("error in (no error)"=w688, "Status"="Device Off", "Module"=w686) -> ("error out"=w698:errorcluster, "Module"=w693:refnum<class "ModuleAdmin.lvclass">)  [unwired: 7 in]
                n127 = Select(t="Start" ("strngStateIn"), s=w696, f=w694) -> (s? t:f=w682:string)
                n128 = call "Enqueue.vi"("EnqueType (Enque)"=enum16{"LossyEnque", "EnqueAtFront", "Enque"}."LossyEnque" ("Enum"), "error in (no error)"=w698, "Message"=w682, "MessageQueue"=w690) -> ("error out"=w697:errorcluster)  [unwired: 6 in, 1 out]
              }
            }
          }
          frame "StartMeas" {
            n129 = call "Enqueue.vi"("EnqueType (Enque)"=enum16{"LossyEnque", "EnqueAtFront", "Enque"}."LossyEnque" ("Enum"), "error in (no error)"=w717, "Message Data"=w711, "Message"="Start" ("strngStateIn"), "MessageQueue"=w714) -> ("error out"=w716:errorcluster)  [unwired: 5 in, 1 out]
          }
          frame "StopMeas" {
            n130 = call "Enqueue.vi"("EnqueType (Enque)"=enum16{"LossyEnque", "EnqueAtFront", "Enque"}."LossyEnque" ("Enum"), "error in (no error)"=w723, "Message"="Stop" ("strngStateIn"), "MessageQueue"=w720) -> ("error out"=w722:errorcluster)  [unwired: 6 in, 1 out]
          }
          frame "PrefDlg" {
            # "Launch the modal Preferences dialog"
            n131 = Preview Queue Element(queue=w724, error in (no error)=w727) -> (element=w725:refnum<class "AcPwrBase.lvclass">, error out=w726:errorcluster)  [unwired: 1 in, 2 out]
            n132 = call-dynamic "PrefDialog.vi"("error in (no error)"=w726, "MyPluginsBase in"=w725) -> ("error out"=w733:errorcluster, "Save As"=w729:bool, "Changed"=w734:bool, "MyPluginsBase out"=w735:refnum<class "AcPwrBase.lvclass">)  [unwired: 6 in]
            n133 = case shown="True" w734 {
              selector: w734 -> [_ w749]
              tunnel: w735 -> [_ w744]
              tunnel: w733 -> [w740 w746]
              tunnel: [w739 w751] -> w732
              tunnel: w731 -> [w738 w752]
              tunnel: [w737 w750] -> w730
              tunnel: w729 -> [_ w745]
              tunnel: w728 -> [_ w748]
              tunnel: w724 -> [_ w747]
              frame False {
                n134 = call "StatusUpdate.vi"("error in (no error)"=w740, "Status"="Preferences Cancelled", "Module"=w738) -> ("error out"=w739:errorcluster, "Module"=w737:refnum<class "ModuleAdmin.lvclass">)  [unwired: 7 in]
              }
              frame True {
                n135 = call-dynamic "ChangeWhileMeasuring.vi"("error in (no error)"=w746, "AcPwrBase in"=w744) -> ("error out"=w742:errorcluster, "InstrumentSettings"=w741:bool, "AcPwrBase out"=w743:refnum<class "AcPwrBase.lvclass">)  [unwired: 6 in, 1 out]
                n136 = case shown="False" w741 {
                  tunnel: w752 -> [w762 w796]
                  tunnel: [w761 w795] -> w751
                  tunnel: [w758 w792] -> w750
                  tunnel: w742 -> [w756 w782]
                  tunnel: w743 -> [w753 w780]
                  tunnel: w749 -> [_ w791]
                  tunnel: w745 -> [w757 w790]
                  tunnel: w748 -> [_ w770]
                  tunnel: w747 -> [w754 w786]
                  frame True {
                    n137 = Lossy Enqueue Element(queue=w754, element=w753, error in (no error)=w756) -> (error out=w755:errorcluster)  [unwired: 3 out]
                    n138 = call "StatusUpdate.vi"("error in (no error)"=w755, "Status"="Preferences Loaded", "Module"=w762) -> ("error out"=w759:errorcluster, "Module"=w760:refnum<class "ModuleAdmin.lvclass">)  [unwired: 7 in]
                    n139 = case shown="True" w757 {
                      tunnel: [w764 w768] -> w761
                      tunnel: w760 -> [w765 w766]
                      tunnel: w759 -> [w764 w767]
                      tunnel: [w765 w766] -> w758
                      frame False {
                      }
                      frame True {
                        n140 = call "ReloadConfigurationFile.vi"("error in (no error)"=w767, "reference In"=w766) -> ("error out"=w768:errorcluster)  [unwired: 9 in]
                      }
                    }
                  }
                  frame False {
                    n141 = call "Dequeue.vi"("PreviewQueue(F)"=TRUE, "error in (no error)"=w782, "MessageQueue"=w770) -> ("error out"=w781:errorcluster, "Message"=w775:string)  [unwired: 4 in, 3 out]
                    n142 = call "CheckonIdle.vi"("MessageQueue"=w770, "OverwriteClass? (F)"=w791, "error in (no error)"=w781, "ChangeOccured? (F)"=w791, "AcPwrBase in"=w780) -> ("Error Out"=w789:errorcluster, "Write?"=w787:bool, "AcPwrBase out"=w788:refnum<class "AcPwrBase.lvclass">)  [unwired: 4 in]
                    n143 = Equal?(x="Run" ("y"), y=w775) -> (x = y?=w772:bool)
                    n144 = case shown="True" w787 {
                      tunnel: w789 -> [w801 w806]
                      tunnel: [w801 w805] -> w784
                      tunnel: w786 -> [_ w804]
                      tunnel: w788 -> [w800 w803]
                      tunnel: [w800 w803] -> w771
                      tunnel: w770 -> [w799 w802]
                      tunnel: [w799 w802] -> w769
                      frame False {
                      }
                      frame True {
                        n145 = Lossy Enqueue Element(queue=w804, element=w803, error in (no error)=w806) -> (error out=w805:errorcluster)  [unwired: 3 out]
                      }
                    }
                    n146 = call-dynamic "ConnectedStatus.vi"("error in (no error)"=w784, "AcPwrBase in"=w771) -> ("error out"=w785:errorcluster, "Any Connections"=w774:bool)  [unwired: 7 in, 1 out]
                    n147 = And(x=w774, y=w772) -> (x .and. y?=w773:bool)
                    n148 = Select(t="Start" ("strngStateIn"), s=w773, f=w775) -> (s? t:f=w776:string)
                    n149 = call "Enqueue.vi"("EnqueType (Enque)"=enum16{"LossyEnque", "EnqueAtFront", "Enque"}."LossyEnque" ("Enum"), "error in (no error)"=w785, "Message"=w776, "MessageQueue"=w769) -> ("error out"=w797:errorcluster)  [unwired: 6 in, 1 out]
                    n150 = call "StatusUpdate.vi"("error in (no error)"=w797, "Status"="Preferences Loaded", "Module"=w796) -> ("error out"=w793:errorcluster, "Module"=w794:refnum<class "ModuleAdmin.lvclass">)  [unwired: 7 in]
                    n151 = case shown="True" w790 {
                      tunnel: [w807 w811] -> w795
                      tunnel: w794 -> [w808 w809]
                      tunnel: w793 -> [w807 w810]
                      tunnel: [w808 w809] -> w792
                      frame False {
                      }
                      frame True {
                        n152 = call "ReloadConfigurationFile.vi"("error in (no error)"=w810, "reference In"=w809) -> ("error out"=w811:errorcluster)  [unwired: 9 in]
                      }
                    }
                  }
                }
              }
            }
          }
          frame "Reset" {
            w822 = TRUE ("btnSet")
            n153 = Preview Queue Element(queue=w816, error in (no error)=w815) -> (queue out=w812:refnum<queue>, element=w823:refnum<class "AcPwrBase.lvclass">, error out=w814:errorcluster)  [unwired: 1 in, 1 out]
            n154 = call "CheckonIdle.vi"("MessageQueue"=w813, "OverwriteClass? (F)"=w822, "error in (no error)"=w814, "ChangeOccured? (F)"=w822, "AcPwrBase in"=w823) -> ("Error Out"=w821:errorcluster, "Write?"=w819:bool, "AcPwrBase out"=w820:refnum<class "AcPwrBase.lvclass">)  [unwired: 4 in]
            n155 = call-dynamic "Reset.vi"("error in (no error)"=w821, "AcPwrBase in"=w820) -> ("error out"=w818:errorcluster, "AcPwrBase out"=w824:refnum<class "AcPwrBase.lvclass">)  [unwired: 8 in]
            n156 = case shown="True" w819 {
              tunnel: w818 -> [w829 w833]
              tunnel: [w829 w832] -> w817
              tunnel: w824 -> [_ w831]
              tunnel: w812 -> [_ w830]
              frame False {
              }
              frame True {
                n157 = Lossy Enqueue Element(queue=w830, element=w831, error in (no error)=w833) -> (error out=w832:errorcluster)  [unwired: 3 out]
              }
            }
            n158 = call "StatusUpdate.vi"("error in (no error)"=w817, "Status"="Device Reset", "Module"=w826) -> ("error out"=w828:errorcluster, "Module"=w825:refnum<class "ModuleAdmin.lvclass">)  [unwired: 7 in]
          }
          frame "Close" {
            w841 = TRUE ("btnSet")
            n159 = Preview Queue Element(queue=w835, error in (no error)=w837) -> (queue out=w834:refnum<queue>, element=w842:refnum<class "AcPwrBase.lvclass">, error out=w836:errorcluster)  [unwired: 1 in, 1 out]
            n160 = call "CheckonIdle.vi"("MessageQueue"=w840, "OverwriteClass? (F)"=w841, "error in (no error)"=w836, "ChangeOccured? (F)"=w841, "AcPwrBase in"=w842) -> ("Error Out"=w845:errorcluster, "Write?"=w843:bool, "AcPwrBase out"=w844:refnum<class "AcPwrBase.lvclass">)  [unwired: 4 in]
            n161 = call-dynamic "Close.vi"("error in (no error)"=w845, "AcPwrBase in"=w844) -> ("error out"=w839:errorcluster, "AcPwrBase out"=w846:refnum<class "AcPwrBase.lvclass">)  [unwired: 8 in]
            n162 = case shown="True" w843 {
              tunnel: w839 -> [w851 w855]
              tunnel: [w851 w854] -> w838
              tunnel: w846 -> [_ w853]
              tunnel: w834 -> [_ w852]
              frame False {
              }
              frame True {
                n163 = Lossy Enqueue Element(queue=w852, element=w853, error in (no error)=w855) -> (error out=w854:errorcluster)  [unwired: 3 out]
              }
            }
            n164 = call "StatusUpdate.vi"("error in (no error)"=w838, "Status"="Device Closed", "Module"=w849) -> ("error out"=w850:errorcluster, "Module"=w848:refnum<class "ModuleAdmin.lvclass">)  [unwired: 7 in]
          }
          frame "Exit" {
            w857 = TRUE
            # "Called by the StopRequest event handler case"
            n165 = control-ref of="This VI"() -> (w867:refnum<vi>)
            n166 = call "Enqueue.vi"("EnqueType (Enque)"=enum16{"LossyEnque", "EnqueAtFront", "Enque"}."LossyEnque" ("Enum"), "error in (no error)"=w864, "Message"="Exit" ("strngStateIn"), "MessageQueue"=w862) -> ("error out"=w863:errorcluster)  [unwired: 6 in, 1 out]
            n167 = call "HandleExit.vi"("error in (no error)"=w863, "VI Refnum"=w867, "StopArgument"=w861, "ModuleAdmin"=w860) -> ("error out"=w868:errorcluster, "Exit via Stop Module Req?"=w865:bool, "WaitForStop?"=w866:bool)  [unwired: 5 in]
            n168 = call <extravilib>:"Write.vi"("element"=w857) -> ("channel"=w856:T5)  [unwired: 1 out]
          }
          frame "Error" {
            # "Handle any errors"
            n169 = property class="ModuleAdmin.lvclass"(reference=w874, error in=w872) -> (reference out=w873:refnum<class "ModuleAdmin.lvclass">, error out=w869:errorcluster, "Accessors:External Launch"=w878:bool, "Accessors:Module ID"=w876:i32)
            n170 = Variant To Data(error in=w869, type=errorcluster {"status"=FALSE, "code"=0, "source"=""} ("error constant"), Variant=w882) -> (data=w877:errorcluster, error out=w880:errorcluster)
            n171 = call "ReportError.vi"("error in (no error)"=w880, "ErrorReported"=w877, "ModuleID"=w876) -> ("error out"=w879:errorcluster)  [unwired: 8 in]
            n172 = case shown="True" w878 {
              tunnel: w879 -> [w887 w891]
              tunnel: w877 -> [w889 _]
              tunnel: [w887 w891] -> w875
              tunnel: [w883 FALSE ("T button?")] -> w870
              frame False {
                w888 = T6 0 items=["no dialog", "OK message", "continue or stop message", "OK message + warnings", "continue/stop + warnings"] ("type of dialog (OK msg:1)")
                # "Stand alone: now, force an exit"
                n173 = call <vilib>:"Simple Error Handler.vi"("type of dialog (OK msg:1)"=w888, "error in (no error)"=w889) -> ("message"=w884:string)  [unwired: 3 in, 4 out]
                n174 = Two Button Dialog(message=w884, 1:"Continue" ("F button name (\"Cancel\")"), 2:"Exit" ("T button name (\"OK\")")) -> (T button?=w883:bool)
              }
              frame True {
                # "Externally launched modules only broadcast the error msg"
              }
            }
            n175 = call <extravilib>:"Write.vi"("element"=w870) -> ("channel"=w871:T5)  [unwired: 1 out]
          }
          frame Default {
            # "Called only if a message was queued and no QMH case was created"
            n176 = property class="ModuleAdmin.lvclass"(reference=w900) -> (reference out=w895:refnum<class "ModuleAdmin.lvclass">, error out=w894:errorcluster, "Accessors:Module ID"=w899:i32, "Accessors:ModuleName"=w896:string)  [unwired: 1 in]
            n177 = call <userlib>:"ModuleName.vi"("Name"=w896, "ModuleID"=w899) -> ("ModuleName"=w898:string)  [unwired: 9 in]
            n178 = xnode "Error Ring"("parameter 0"=w897, "parameter 1"=w898) -> ("error out"=w893:errorcluster)
            n179 = Merge Errors(w894, w893) -> (w892:errorcluster)
          }
        }
        n180 = call "ErrorHandler.vi"("error in (no error)"=w341, "MessageQueue"=w339) -> ("error out"=w338:errorcluster)  [unwired: 8 in, 1 out]
      }
      n181 = while {
        tunnel: w60 -> [w78]
        tunnel: [w75] -> w59
        tunnel: w58 -> [w81]
        tunnel: w57 -> [w79]
        tunnel: w55 -> [w74]
        tunnel: [w74] -> w56
        tunnel: w54 -> [w71]
        stop <- w82 stop-if-true
        # "Measurement Acquisition Loop"
        n182 = call "Dequeue.vi"("PreviewQueue(F)"=TRUE, "error in (no error)"=w78, "MessageQueue"=w74) -> ("error out"=w77:errorcluster, "Message Data"=w70:variant, "Message"=w76:string, "MessageQueue"=w73:refnum<queue>)  [unwired: 4 in, 1 out]
        n183 = case shown="\"Run\"" w76 {
          tunnel: [_ _ _ _ TRUE] -> w82
          tunnel: w77 -> [w83 w89 w111 w148 w155]
          tunnel: [w84 w96 w113 w150 w155] -> w80
          tunnel: w81 -> [_ w93 w114 w146 _]
          tunnel: w73 -> [_ w95 w112 w149 _]
          tunnel: w71 -> [_ w92 w110 w145 _]
          tunnel: w70 -> [_ w88 _ _ _]
          frame "Idle", Default {
            n184 = flat-sequence {
              tunnel: [w85] -> w84
              tunnel: w83 -> [w85]
              frame #0 {
                n185 = Wait (ms)(milliseconds to wait=u32 50) -> ()  [unwired: 1 out]
              }
            }
          }
          frame "Start" {
            n186 = Preview Queue Element(queue=w92, error in (no error)=w89) -> (element=w87:refnum<class "AcPwrBase.lvclass">, error out=w94:errorcluster)  [unwired: 1 in, 2 out]
            n187 = call-dynamic "StartMeas.vi"("error in (no error)"=w94, "Variant"=w88, "AcPwrBase in"=w87) -> ("error out"=w98:errorcluster)  [unwired: 7 in, 1 out]
            n188 = call "StatusUpdate.vi"("error in (no error)"=w98, "Status"="Measurements Started", "Module"=w93) -> ("error out"=w97:errorcluster)  [unwired: 7 in, 1 out]
            n189 = call "Enqueue.vi"("EnqueType (Enque)"=enum16{"LossyEnque", "EnqueAtFront", "Enque"}."LossyEnque" ("Enum"), "error in (no error)"=w97, "Message"="Run" ("strngStateIn"), "MessageQueue"=w95) -> ("error out"=w96:errorcluster)  [unwired: 6 in, 1 out]
          }
          frame "Run" {
            n190 = flat-sequence {
              tunnel: w110 -> [w116]
              tunnel: w111 -> [w117]
              tunnel: w112 -> [w118]
              tunnel: w114 -> [w119]
              tunnel: [w119] -> w108
              tunnel: [w118] -> w107
              tunnel: [w117] -> w106
              tunnel: [w116] -> w105
              tunnel: [w115] -> w103
              tunnel: [w130] -> w109
              tunnel: w108 -> [w132]
              tunnel: w107 -> [w127]
              tunnel: w106 -> [w125]
              tunnel: w105 -> [w124]
              tunnel: [w120] -> w104
              tunnel: w103 -> [w120]
              tunnel: [w142] -> w113
              tunnel: w109 -> [w142]
              tunnel: w104 -> [w141]
              tunnel: [w141] -> w102
              tunnel: [w140] -> w101
              frame #0 {
                n191 = Tick Count (ms)() -> (millisecond timer value=w115:u32)
              }
              frame #1 {
                n192 = Preview Queue Element(queue=w124, error in (no error)=w125) -> (queue out=w121:refnum<queue>, element=w133:refnum<class "AcPwrBase.lvclass">, error out=w126:errorcluster)  [unwired: 1 in, 1 out]
                n193 = call-dynamic "RunMeas.vi"("error in (no error)"=w126, "AcPwrBase in"=w133) -> ("error out"=w129:errorcluster, "variant"=w128:variant)  [unwired: 7 in, 1 out]
                n194 = call "Measurements.vi"("error in (no error)"=w129, "variant"=w128, "Module"=w132) -> ("error out"=w131:errorcluster)  [unwired: 8 in]
                n195 = case shown="No Error" w131 {
                  selector: w131 -> [w134 w135]
                  tunnel: [w134 w139] -> w130
                  tunnel: w127 -> [_ w138]
                  tunnel: enum16{"LossyEnque", "EnqueAtFront", "Enque"}."LossyEnque" ("Enum") -> [_ w136]
                  tunnel: "Stop" ("strngStateIn") -> [_ w137]
                  tunnel: w121 -> [_ _]
                  frame No Error {
                  }
                  frame Error {
                    n196 = call "Enqueue.vi"("EnqueType (Enque)"=w136, "error in (no error)"=w135, "Message"=w137, "MessageQueue"=w138) -> ("error out"=w139:errorcluster)  [unwired: 6 in, 1 out]
                  }
                }
              }
              frame #2 {
                n197 = Tick Count (ms)() -> (millisecond timer value=w140:u32)
              }
            }
            n198 = Subtract(x=w101, y=w102) -> (x-y=→"RunTime(ms)":u32)
          }
          frame "Stop" {
            n199 = Preview Queue Element(queue=w145, error in (no error)=w148) -> (element=w154:refnum<class "AcPwrBase.lvclass">, error out=w147:errorcluster)  [unwired: 1 in, 2 out]
            n200 = call-dynamic "StopMeas.vi"("error in (no error)"=w147, "AcPwrBase in"=w154) -> ("error out"=w152:errorcluster)  [unwired: 8 in, 1 out]
            n201 = call "StatusUpdate.vi"("error in (no error)"=w152, "Status"="Measurements Stopped", "Module"=w146) -> ("error out"=w151:errorcluster)  [unwired: 7 in, 1 out]
            n202 = call "Enqueue.vi"("EnqueType (Enque)"=enum16{"LossyEnque", "EnqueAtFront", "Enque"}."LossyEnque" ("Enum"), "error in (no error)"=w151, "Message"="Idle" ("strngStateIn"), "MessageQueue"=w149) -> ("error out"=w150:errorcluster)  [unwired: 6 in, 1 out]
          }
          frame "Exit" {
          }
        }
        n203 = call "ErrorHandler.vi"("error in (no error)"=w80, "MessageQueue"=w79) -> ("error out"=w75:errorcluster)  [unwired: 8 in, 1 out]
      }
      n204 = while {
        tunnel: w57 -> [w159]
        shift-right: [w163] -> w62
        shift-left: w67 -> [w164]
        tunnel: w58 -> [w162]
        tunnel: [w160] -> w63
        tunnel: w52 -> [w157]
        stop <- w165 stop-if-true
        # "Event Handler Loop"
        n205 = event shown="[1] Timeout" {
          selector: w164 -> [_ _ _ _ _ _ _ _ _ _ _ _ _ _ _ _ _]
          dyn-events: [_ _ _ _ _ _ _ _ _ _ _ _ _ _ _ _ _] -> w163
          timeout: 100 -> [_ _ _ _ _ _ _ _ _ _ _ _ _ _ _ _ _]
          tunnel: w159 -> [w178 _ w185 w202 w213 w222 w232 w239 w247 w256 w266 w276 w285 w294 w303 w311 w322]
          tunnel: [TRUE w179 w184 _ _ _ _ _ _ _ _ _ _ _ _ _ _] -> w165
          tunnel: w162 -> [w172 _ w188 w206 w212 w226 w235 w243 w251 w260 w270 w279 w288 w296 w305 w315 w321]
          tunnel: [w176 errorcluster {"status"=FALSE, "code"=0, "source"=""} ("error out") w183 w203 w211 w223 w231 w240 w248 w257 w267 w275 w283 w295 w304 w312 w323] -> w161
          tunnel: w157 -> [_ w180 _ _ _ _ _ _ _ _ _ _ _ _ _ _ _]
          event Panel Close? {
            # "Hide on external launch"
            # "Discard the event so the QMH can complete"
            # "Called from another module or the QMH"
            n206 = event-data() -> ()  [unwired: 1 in, 1 out]
            n207 = property class="ModuleAdmin.lvclass"(reference=w172) -> ("Accessors:External Launch"=w167:bool)  [unwired: 1 in, 2 out]
            n208 = Bundle By Name(cluster=T3 {"Exit via Stop Module Req?"=FALSE, "Wait for Module to stop?"=FALSE, "ModuleAdmin"=refnum} ("Stop Argument"), "Wait for Module to stop?"=FALSE, "Exit via Stop Module Req?"=TRUE) -> (w173:T3)
            n209 = Select(t="HidePanel", s=w167, f="Exit" ("Message")) -> (s? t:f=w169:string)
            n210 = call "Enqueue.vi"("Message Data"=w173, "Message"=w169, "MessageQueue"=w178) -> ("error out"=w176:errorcluster)  [unwired: 7 in, 1 out]
            n211 = event-data("Discard?"=TRUE) -> ()  [unwired: 1 in, 1 out]
          }
          event Timeout {
            n212 = event-data() -> ()  [unwired: 1 in, 1 out]
            n213 = call <extravilib>:"Read.vi"("channel"=w180) -> ("element"=w179:bool)  [unwired: 1 in, 1 out]
          }
          event User Event {
            # "Called from another module or the QMH"
            n214 = event-data() -> ("ModuleID"=w186:i32, "Data"=w182:variant)  [unwired: 1 in]
            n215 = call <userlib>:"AddressedToThisModule.vi"("ModuleID"=w186, "ModuleAdmin"=w188) -> ("AddressedToThisInstance?"=w187:bool)  [unwired: 8 in, 1 out]
            n216 = case shown="True" w187 {
              tunnel: w185 -> [_ w192]
              tunnel: [FALSE TRUE] -> w184
              tunnel: [_ w196] -> w183
              tunnel: w182 -> [_ w190]
              frame False {
                # "The stop request was for a different module"
              }
              frame True {
                # "The stop request was for this module"
                n217 = call "Enqueue.vi"("Message"="DeviceOff", "MessageQueue"=w192) -> ("error out"=w194:errorcluster, "MessageQueue"=w193:refnum<queue>)  [unwired: 8 in]
                n218 = call "Enqueue.vi"("error in (no error)"=w194, "Message"="Close", "MessageQueue"=w193) -> ("error out"=w197:errorcluster, "MessageQueue"=w195:refnum<queue>)  [unwired: 7 in]
                n219 = call "Enqueue.vi"("error in (no error)"=w197, "Message Data"=w190, "Message"="Exit", "MessageQueue"=w195) -> ("error out"=w196:errorcluster)  [unwired: 6 in, 1 out]
              }
            }
          }
          event User Event {
            n220 = event-data() -> ("ModuleID"=w205:i32, "Data"=w201:variant)  [unwired: 1 in]
            n221 = call <userlib>:"AddressedToThisModule.vi"("ModuleID"=w205, "ModuleAdmin"=w206) -> ("AddressedToThisInstance?"=w204:bool)  [unwired: 8 in, 1 out]
            n222 = case shown="True" w204 {
              tunnel: [_ w207] -> w203
              tunnel: w202 -> [_ w210]
              tunnel: w201 -> [_ w208]
              frame False {
              }
              frame True {
                n223 = call "Enqueue.vi"("Message Data"=w208, "Message"="ShowPanel", "MessageQueue"=w210) -> ("error out"=w207:errorcluster)  [unwired: 7 in, 1 out]
              }
            }
          }
          event User Event {
            n224 = event-data() -> ("ModuleID"=w214:i32, "Data"=w215:variant)  [unwired: 1 in]
            n225 = call <userlib>:"AddressedToThisModule.vi"("ModuleID"=w214, "ModuleAdmin"=w212) -> ("AddressedToThisInstance?"=w216:bool)  [unwired: 8 in, 1 out]
            n226 = case shown="True" w216 {
              tunnel: w213 -> [_ w220]
              tunnel: [_ w219] -> w211
              tunnel: w215 -> [_ w217]
              frame False {
                (unwired) FALSE
                # "The stop request was for a different module"
              }
              frame True {
                # "The stop request was for this module"
                n227 = call "Enqueue.vi"("Message Data"=w217, "Message"="GetPathToINI", "MessageQueue"=w220) -> ("error out"=w219:errorcluster)  [unwired: 7 in, 1 out]
              }
            }
          }
          event User Event {
            n228 = event-data() -> ("ModuleID"=w225:i32, "Data"=w221:variant)  [unwired: 1 in]
            n229 = call <userlib>:"AddressedToThisModule.vi"("ModuleID"=w225, "ModuleAdmin"=w226) -> ("AddressedToThisInstance?"=w224:bool)  [unwired: 8 in, 1 out]
            n230 = case shown="True" w224 {
              tunnel: [_ w227] -> w223
              tunnel: w222 -> [_ w230]
              tunnel: w221 -> [_ w228]
              frame False {
              }
              frame True {
                n231 = call "Enqueue.vi"("Message Data"=w228, "Message"="LoadPlugin", "MessageQueue"=w230) -> ("error out"=w227:errorcluster)  [unwired: 7 in, 1 out]
              }
            }
          }
          event User Event {
            n232 = event-data() -> ("ModuleID"=w234:i32)  [unwired: 1 in]
            n233 = call <userlib>:"AddressedToThisModule.vi"("ModuleID"=w234, "ModuleAdmin"=w235) -> ("AddressedToThisInstance?"=w233:bool)  [unwired: 8 in, 1 out]
            n234 = case shown="True" w233 {
              tunnel: w232 -> [_ w237]
              tunnel: [_ w236] -> w231
              frame False {
              }
              frame True {
                n235 = call "Enqueue.vi"("Message"="InitAcPower", "MessageQueue"=w237) -> ("error out"=w236:errorcluster)  [unwired: 8 in, 1 out]
              }
            }
          }
          event User Event {
            n236 = event-data() -> ("ModuleID"=w242:i32)  [unwired: 1 in]
            n237 = call <userlib>:"AddressedToThisModule.vi"("ModuleID"=w242, "ModuleAdmin"=w243) -> ("AddressedToThisInstance?"=w241:bool)  [unwired: 8 in, 1 out]
            n238 = case shown="True" w241 {
              tunnel: [_ w244] -> w240
              tunnel: w239 -> [_ w246]
              frame False {
              }
              frame True {
                n239 = call "Enqueue.vi"("Message"="PrefDlg", "MessageQueue"=w246) -> ("error out"=w244:errorcluster)  [unwired: 8 in, 1 out]
              }
            }
          }
          event User Event {
            n240 = event-data() -> ("ModuleID"=w250:i32)  [unwired: 1 in]
            n241 = call <userlib>:"AddressedToThisModule.vi"("ModuleID"=w250, "ModuleAdmin"=w251) -> ("AddressedToThisInstance?"=w249:bool)  [unwired: 8 in, 1 out]
            n242 = case shown="True" w249 {
              tunnel: [_ w254] -> w248
              tunnel: w247 -> [_ w252]
              frame False {
              }
              frame True {
                n243 = call "Enqueue.vi"("Message"="ConfigDevice", "MessageQueue"=w252) -> ("error out"=w254:errorcluster)  [unwired: 8 in, 1 out]
              }
            }
          }
          event User Event {
            n244 = event-data() -> ("ModuleID"=w259:i32, "Data"=w255:variant)  [unwired: 1 in]
            n245 = call <userlib>:"AddressedToThisModule.vi"("ModuleID"=w259, "ModuleAdmin"=w260) -> ("AddressedToThisInstance?"=w258:bool)  [unwired: 8 in, 1 out]
            n246 = case shown="True" w258 {
              tunnel: [_ w262] -> w257
              tunnel: w256 -> [_ w263]
              tunnel: w255 -> [_ w261]
              frame False {
              }
              frame True {
                n247 = call "Enqueue.vi"("Message Data"=w261, "Message"="GetSettings", "MessageQueue"=w263) -> ("error out"=w262:errorcluster)  [unwired: 7 in, 1 out]
              }
            }
          }
          event User Event {
            n248 = event-data() -> ("ModuleID"=w269:i32, "Data"=w265:variant)  [unwired: 1 in]
            n249 = call <userlib>:"AddressedToThisModule.vi"("ModuleID"=w269, "ModuleAdmin"=w270) -> ("AddressedToThisInstance?"=w268:bool)  [unwired: 8 in, 1 out]
            n250 = case shown="True" w268 {
              tunnel: [_ w271] -> w267
              tunnel: w266 -> [_ w273]
              tunnel: w265 -> [_ w272]
              frame False {
              }
              frame True {
                n251 = call "Enqueue.vi"("Message Data"=w272, "Message"="SetSettings", "MessageQueue"=w273) -> ("error out"=w271:errorcluster)  [unwired: 7 in, 1 out]
              }
            }
          }
          event User Event {
            n252 = event-data() -> ("ModuleID"=w278:i32)  [unwired: 1 in]
            n253 = call <userlib>:"AddressedToThisModule.vi"("ModuleID"=w278, "ModuleAdmin"=w279) -> ("AddressedToThisInstance?"=w277:bool)  [unwired: 8 in, 1 out]
            n254 = case shown="True" w277 {
              tunnel: w276 -> [_ w281]
              tunnel: [_ w280] -> w275
              frame False {
              }
              frame True {
                n255 = call "Enqueue.vi"("Message"="DeviceOn", "MessageQueue"=w281) -> ("error out"=w280:errorcluster)  [unwired: 8 in, 1 out]
              }
            }
          }
          event User Event {
            n256 = event-data() -> ("ModuleID"=w287:i32, "Data"=w284:variant)  [unwired: 1 in]
            n257 = call <userlib>:"AddressedToThisModule.vi"("ModuleID"=w287, "ModuleAdmin"=w288) -> ("AddressedToThisInstance?"=w286:bool)  [unwired: 8 in, 1 out]
            n258 = case shown="True" w286 {
              tunnel: w285 -> [_ w291]
              tunnel: w284 -> [_ w290]
              tunnel: [_ w289] -> w283
              frame False {
              }
              frame True {
                n259 = call "Enqueue.vi"("Message Data"=w290, "Message"="DeviceOff", "MessageQueue"=w291) -> ("error out"=w289:errorcluster)  [unwired: 7 in, 1 out]
              }
            }
          }
          event User Event {
            n260 = event-data() -> ("ModuleID"=w298:i32, "Data"=w293:variant)  [unwired: 1 in]
            n261 = call <userlib>:"AddressedToThisModule.vi"("ModuleID"=w298, "ModuleAdmin"=w296) -> ("AddressedToThisInstance?"=w297:bool)  [unwired: 8 in, 1 out]
            n262 = case shown="True" w297 {
              tunnel: [_ w301] -> w295
              tunnel: w294 -> [_ w300]
              tunnel: w293 -> [_ w299]
              frame False {
              }
              frame True {
                n263 = call "Enqueue.vi"("Message Data"=w299, "Message"="StartMeas", "MessageQueue"=w300) -> ("error out"=w301:errorcluster)  [unwired: 7 in, 1 out]
              }
            }
          }
          event User Event {
            n264 = event-data() -> ("ModuleID"=w306:i32)  [unwired: 1 in]
            n265 = call <userlib>:"AddressedToThisModule.vi"("ModuleID"=w306, "ModuleAdmin"=w305) -> ("AddressedToThisInstance?"=w307:bool)  [unwired: 8 in, 1 out]
            n266 = case shown="True" w307 {
              tunnel: [_ w308] -> w304
              tunnel: w303 -> [_ w309]
              frame False {
              }
              frame True {
                n267 = call "Enqueue.vi"("Message"="StopMeas", "MessageQueue"=w309) -> ("error out"=w308:errorcluster)  [unwired: 8 in, 1 out]
              }
            }
          }
          event User Event {
            n268 = event-data() -> ("ModuleID"=w314:i32)  [unwired: 1 in]
            n269 = call <userlib>:"AddressedToThisModule.vi"("ModuleID"=w314, "ModuleAdmin"=w315) -> ("AddressedToThisInstance?"=w313:bool)  [unwired: 8 in, 1 out]
            n270 = case shown="True" w313 {
              tunnel: [_ w318] -> w312
              tunnel: w311 -> [_ w316]
              frame False {
              }
              frame True {
                n271 = call "Enqueue.vi"("Message"="Reset", "MessageQueue"=w316) -> ("error out"=w318:errorcluster)  [unwired: 8 in, 1 out]
              }
            }
          }
          event User Event {
            n272 = event-data() -> ("ModuleID"=w320:i32)  [unwired: 1 in]
            n273 = call <userlib>:"AddressedToThisModule.vi"("ModuleID"=w320, "ModuleAdmin"=w321) -> ("AddressedToThisInstance?"=w319:bool)  [unwired: 8 in, 1 out]
            n274 = case shown="True" w319 {
              tunnel: [_ w324] -> w323
              tunnel: w322 -> [_ w328]
              frame False {
              }
              frame True {
                n275 = disable-structure shown="Enabled" {
                  disable-tunnel: "DeviceOff" ("Message") -> [w333 _]
                  disable-tunnel: w328 -> [w332 w334]
                  disable-tunnel: [w331 _] -> w327
                  disable-tunnel: [w330 w334] -> w326
                  frame Disabled {
                    n276 = call "Enqueue.vi"("Message"=w333, "MessageQueue"=w332) -> ("error out"=w331:errorcluster, "MessageQueue"=w330:refnum<queue>)  [unwired: 8 in]
                  }
                  frame Enabled {
                  }
                }
                n277 = call "Enqueue.vi"("error in (no error)"=w327, "Message"="Close", "MessageQueue"=w326) -> ("error out"=w324:errorcluster)  [unwired: 7 in, 1 out]
              }
            }
          }
        }
        n278 = call "ErrorHandler.vi"("error in (no error)"=w161, "MessageQueue"=w159) -> ("error out"=w160:errorcluster)  [unwired: 8 in, 1 out]
      }
    }
    frame Error {
      n279 = property class="ModuleAdmin.lvclass"(reference=w918) -> (reference out=w917:refnum<class "ModuleAdmin.lvclass">, "Accessors:CloneRegRef"=w916:refnum<data-value>, "Accessors:Module ID"=w915:i32)  [unwired: 1 in, 1 out]
      n280 = call <userlib>:"Remove.vi"("Module ID"=w915, "CloneRegRef"=w916) -> ("error out"=w919:errorcluster)  [unwired: 7 in, 2 out]
      n281 = flat-sequence {
        tunnel: w920 -> [w923]
        tunnel: w919 -> [_]
        tunnel: [w921] -> w909
        frame #0 {
          w922 = T6 2 items=["no dialog", "OK message", "continue or stop message", "OK message + warnings", "continue/stop + warnings"] ("type of dialog (OK msg:1)")
          n282 = call <vilib>:"Simple Error Handler.vi"("type of dialog (OK msg:1)"=w922, "error in (no error)"=w923) -> ("error out"=w921:errorcluster)  [unwired: 3 in, 4 out]
        }
      }
    }
  }
  n283 = call "DestroyClone.vi"("error in (no error)"=w1, "Exit via Stop Module Req?"=w41, "Wait for Module to stop?"=w42, "ModuleAdmin"=w2) -> ("error out"=w43:errorcluster, "External Launch"=w40:bool)  [unwired: 5 in, 1 out]
  n284 = Unregister For Events(event registration refnum=w38, error in=w39) -> (error out=w36:errorcluster)
  n285 = Release Queue(queue=w35, force destroy? (F)=w19, error in (no error)=w43) -> (error out=w27:errorcluster)  [unwired: 2 out]
  n286 = Release Queue(queue=w26, force destroy? (F)=w19, error in (no error)=w27) -> (error out=w18:errorcluster)  [unwired: 2 out]
  n287 = Release Queue(queue=w16, force destroy? (F)=w19, error in (no error)=w18) -> (error out=w17:errorcluster)  [unwired: 2 out]
  n288 = Merge Errors(w36, w17, w29) -> (w37:errorcluster)
  "error out" <- w37
  n289 = case shown="True" w40 {
    tunnel: w37 -> [_ w925]
    frame False {
    }
    frame True {
      n290 = control-ref of="This VI"() -> (w924:refnum<vi>)
      n291 = case shown="Error" w925 {
        tunnel: w924 -> [w927 w929]
        tunnel: [w926 w928] -> _
        frame No Error {
          n292 = invoke class="VI" method="FP.Close"(reference=w927) -> (error out=w926:errorcluster)  [unwired: 2 in, 2 out]
        }
        frame Error {
          n293 = invoke class="VI" method="FP.Open"(reference=w929, "Activate"=TRUE ("Activate?")) -> (error out=w928:errorcluster)  [unwired: 3 in, 4 out]
        }
      }
    }
  }
